vi "External_Move.vi"(8 "error in (no error)":errorcluster, 11 "Arduino_Stepper_UI in":refnum<class "Arduino_Stepper_UI.lvclass">) -> (0 "error out":errorcluster, 3 "Arduino_Stepper_UI out":refnum<class "Arduino_Stepper_UI.lvclass">)   [LabVIEW 2023, in "Arduino_TranslationStage_UI.lvlib" / "Arduino_Stepper_UI.lvclass"]
uses:
  Arduino_Stepper_UI.lvclass
  Arduino_Stepper_UI.lvclass/Arduino_Stepper_UI.ctl
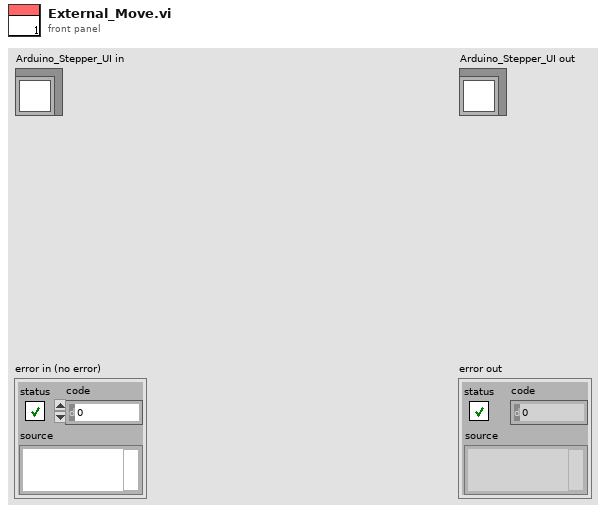
[diagram p1: front panel]
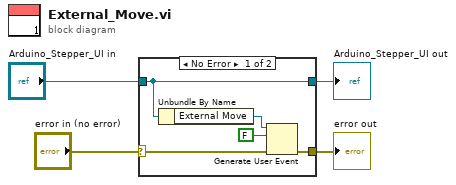
[diagram p0: block diagram]
diagram:
  n1 = case shown="No Error" "error in (no error)" {
    selector: "error in (no error)" -> [w7 w11]
    tunnel: [w6 w11] -> w3
    tunnel: [w9 w10] -> w1
    tunnel: "Arduino_Stepper_UI in" -> [w9 w10]
    frame No Error {
      n2 = Unbundle By Name(w9) -> ("External Move"=w8:refnum<user-event>)
      n3 = Generate User Event(user event=w8, event data cluster=FALSE ("event data"), error in=w7) -> (error out=w6:errorcluster)  [unwired: 1 in, 1 out]
    }
    frame Error {
    }
  }
  "error out" <- w3
  "Arduino_Stepper_UI out" <- w1
